vi "Create.vi"(8 "ErrorArray":errorcluster[](array[cluster]), 10 "name or relative path":string="PARTF\\PARTF.ini") -> (0 "ErrorArray":errorcluster[](array[cluster]), 3 "Ref out":refnum<class "Config.lvclass">)   [LabVIEW 2014, in "Config_class.lvlib" / "Config.lvclass"]
uses:
  Config.lvclass
  <vilib>/Utility/sysdir.llb/System Directory Type.ctl
  Typedefs/RootDir.ctl
  Typedefs/Logging.ctl
  Typedefs/eLogLvl.ctl
  Config.lvclass/Config.ctl
  Accessors/Write ConfigFilePath.vi
  Accessors/Write Logging.vi
  Accessors/Write Root Directory.vi
  <vilib>/Utility/config.llb/NI_LVConfig.lvlib
  <userlib>/NIST/NISTErrorLib/NISTErrorLib.lvlib
panel:
  out "before substring":string
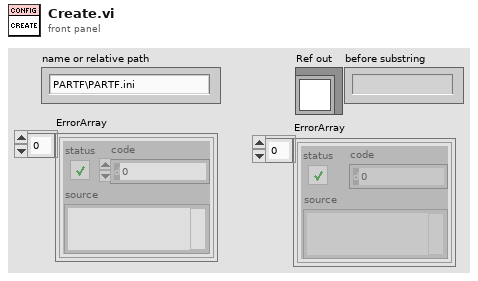
[diagram p1: front panel]
types:
  T1 = typedef "System Directory Type.ctl" = i32
  T2 = typedef "Config_class.lvlib/Config.lvclass/eLogLvl.ctl" = enum16{"Normal", "Verbose", "None"}
  T3 = typedef "Config_class.lvlib/Config.lvclass/Logging.ctl" = cluster{"eLogLvl":T2, "Log File Path":path, "btnLogFile":bool}
  T4 = typedef "Config_class.lvlib/Config.lvclass/RootDir.ctl" = cluster{"pathRootDir":path, "btnOutPath":bool, "OutDir":string, "btnOpenOutputDir":bool, "ScriptDir":string, "btnOpenScriptDir":bool, "TestDir":string, "btnOpenTestDir":bool}
  T5 = cluster{"pathRootDir":path, "OutDir":string, "ScriptDir":string, "TestDir":string}
  T6 = typedef "NI_LVConfig.lvlib/Config Data RefNum.ctl" = refnum<k1>
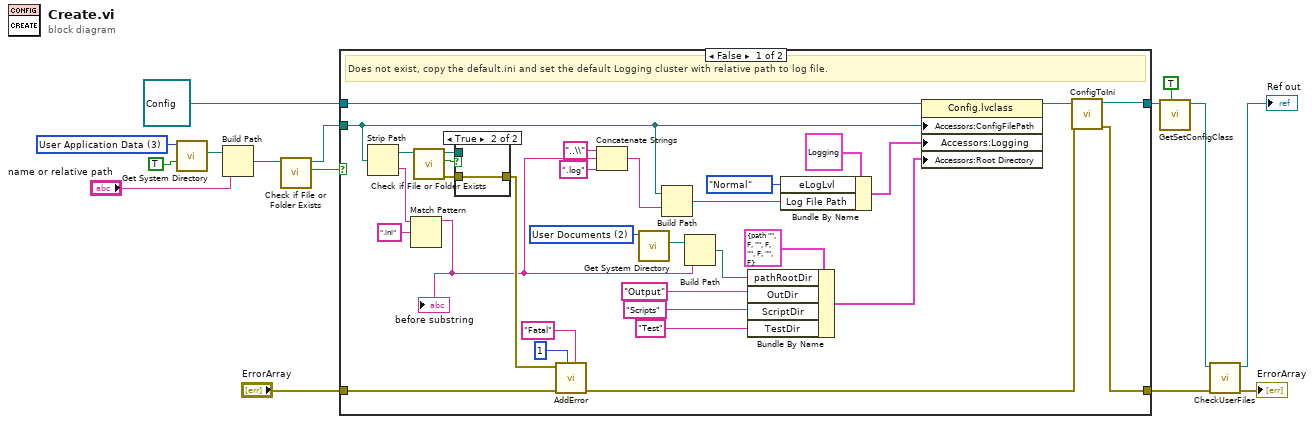
[diagram p0: block diagram]
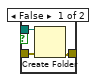
[diagram p2: hidden frame]
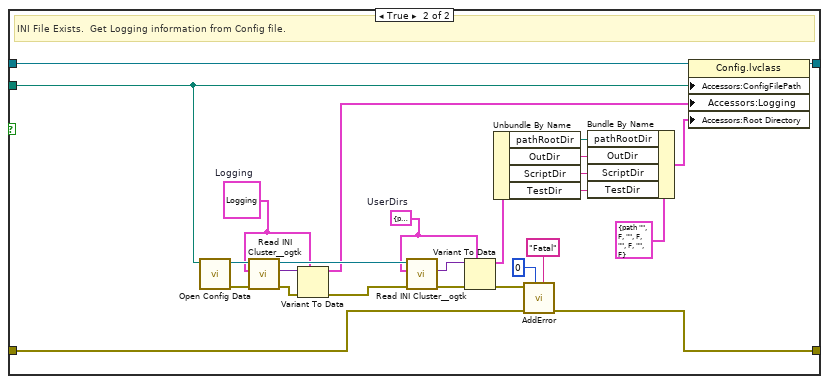
[diagram p3: hidden frame]
diagram:
  w15 = T1 3 items=["User Home"=0, "User Desktop"=1, "User Documents"=2, "User Application Data"=3, "User Preferences"=4, "User Temporary"=5, "Public Documents"=6, "Public Application Data"=7, "Public Preferences"=8, "Public Cache"=13, "System Core Libraries"=9, "System Installed Libraries"=10, "Application Files"=11, "Boot Volume Root"=12] ("system directory type")
  n1 = call <vilib>:"Get System Directory.vi"("create directory if not found? (F)"=TRUE, "system directory type"=w15) -> ("system directory"=w7:path)  [unwired: 9 in]
  n2 = Build Path(base path=w7, name or relative path="name or relative path") -> (appended path=w11:path)
  n3 = call <vilib>:"Check if File or Folder Exists.vi"("path"=w11) -> ("file or folder exists?"=w12:bool, "dup path"=w8:path)  [unwired: 8 in, 1 out]
  n4 = case shown="False" w12 {
    tunnel: w8 -> [w22 w67]
    tunnel: refnum<class "Config.lvclass"> refnum ("Framework.lvlib:Config.lvclass") -> [w47 w77]
    tunnel: [w33 w68] -> w2
    tunnel: "ErrorArray" -> [w31 w64]
    tunnel: [w34 w63] -> w1
    frame False {
      w46 = T1 2 items=["User Home"=0, "User Desktop"=1, "User Documents"=2, "User Application Data"=3, "User Preferences"=4, "User Temporary"=5, "Public Documents"=6, "Public Application Data"=7, "Public Preferences"=8, "Public Cache"=13, "System Core Libraries"=9, "System Installed Libraries"=10, "Application Files"=11, "Boot Volume Root"=12] ("system directory type")
      # "Does not exist, copy the default.ini and set the default Logging cluster with relative path to log file."
      n5 = Strip Path(path=w22) -> (stripped path=w26:path, name=w21:string)
      n6 = Match Pattern(string=w21, regular expression=".ini") -> (before substring=w16:string)  [unwired: 1 in, 3 out]
      "before substring" <- w16
      n7 = call <vilib>:"Check if File or Folder Exists.vi"("path"=w26) -> ("error out"=w23:errorcluster, "file or folder exists?"=w25:bool, "dup path"=w24:path)  [unwired: 8 in]
      n8 = case shown="True" w25 {
        tunnel: [w50 w51] -> w29
        tunnel: w24 -> [w49 _]
        tunnel: w23 -> [w48 w51]
        frame False {
          n9 = Create Folder(path (use dialog)=w49, error in=w48) -> (error out=w50:errorcluster)  [unwired: 1 in, 2 out]
        }
        frame True {
        }
      }
      n10 = call <userlib>:"AddError.vi"("Severity"="Fatal", "Priority"=u8 1, "ErrorArray"=w31, "error in (no error)"=w29) -> ("ErrorArray"=w30:errorcluster[])  [unwired: 6 in, 1 out]
      n11 = Concatenate Strings("..\\" ("string"), w16, ".log" ("string")) -> (w18:string)
      n12 = call <vilib>:"Get System Directory.vi"("system directory type"=w46) -> ("system directory"=w45:path)  [unwired: 10 in]
      n13 = Build Path(base path=w22, name or relative path=w18) -> (appended path=w38:path)
      n14 = Build Path(base path=w45, name or relative path=w16) -> (appended path=w43:path)
      n15 = Bundle By Name(cluster=T4 {"pathRootDir"=path "", "btnOutPath"=FALSE, "OutDir"="", "btnOpenOutputDir"=FALSE, "ScriptDir"="", "btnOpenScriptDir"=FALSE, "TestDir"="", "btnOpenTestDir"=FALSE} ("PARTF Root Directory"), "pathRootDir"=w43, "OutDir"="Output", "ScriptDir"="Scripts", "TestDir"="Test" ("ScriptDir")) -> (w40:T4)
      n16 = Bundle By Name(cluster=T3 {"eLogLvl"=enum."Normal", "Log File Path"=path "C:/Users/gra1/AppData/Local/Framework/Framework.log", "btnLogFile"=FALSE} ("Logging"), "eLogLvl"=eLogLvl."Normal", "Log File Path"=w38) -> (w36:T3)
      n17 = property class="Config.lvclass"(reference=w47, "Accessors:ConfigFilePath"=w22, "Accessors:Logging"=w36, "Accessors:Root Directory"=w40) -> (reference out=w35:refnum<class "Config.lvclass">)  [unwired: 1 in, 1 out]
      n18 = call "ConfigToIni.vi"("Error In"=w30, "ConfigRef"=w35) -> ("Error Out"=w34:errorcluster[], "ConfigRef"=w33:refnum<class "Config.lvclass">)  [unwired: 8 in]
    }
    frame True {
      w60 = T3 {"eLogLvl"=enum."Normal", "Log File Path"=path "C:/Users/gra1/AppData/Local/Framework/Framework.log", "btnLogFile"=FALSE}  # Logging
      w61 = T5 {"pathRootDir"=path "", "OutDir"="", "ScriptDir"="", "TestDir"=""}  # UserDirs
      # "INI File Exists.  Get Logging information from Config file."
      n19 = call <vilib>:"Open Config Data.vi"("configuration file path"=w67) -> ("error out"=w76:errorcluster, "refnum"=w75:T6)  [unwired: 8 in, 1 out]
      n20 = call <userlib>:"Read INI Cluster__ogtk.vi"("error in (no error)"=w76, "INI Fomatted Cluster Type"=w60, "refnum"=w75) -> ("error out"=w74:errorcluster, "INI Fomatted Cluster"=w73:variant, "dup refnum"=w72:T6)  [unwired: 4 in, 2 out]
      n21 = Variant To Data(error in=w74, type=w60, Variant=w73) -> (data=w59:T3, error out=w71:errorcluster)
      n22 = call <userlib>:"Read INI Cluster__ogtk.vi"("error in (no error)"=w71, "INI Fomatted Cluster Type"=w61, "refnum"=w72) -> ("error out"=w70:errorcluster, "INI Fomatted Cluster"=w69:variant)  [unwired: 4 in, 3 out]
      n23 = Variant To Data(error in=w70, type=w61, Variant=w69) -> (data=w58:T5, error out=w62:errorcluster)
      n24 = Unbundle By Name(w58) -> ("pathRootDir"=w56:path, "OutDir"=w55:string, "ScriptDir"=w54:string, "TestDir"=w53:string)
      n25 = call <userlib>:"AddError.vi"("Severity"="Fatal", "Priority"=u8 0, "ErrorArray"=w64, "error in (no error)"=w62) -> ("ErrorArray"=w63:errorcluster[])  [unwired: 6 in, 1 out]
      n26 = Bundle By Name(cluster=T4 {"pathRootDir"=path "", "btnOutPath"=FALSE, "OutDir"="", "btnOpenOutputDir"=FALSE, "ScriptDir"="", "btnOpenScriptDir"=FALSE, "TestDir"="", "btnOpenTestDir"=FALSE} ("PARTF Root Directory"), "pathRootDir"=w56, "OutDir"=w55, "ScriptDir"=w54, "TestDir"=w53) -> (w52:T4)
      n27 = property class="Config.lvclass"(reference=w77, "Accessors:ConfigFilePath"=w67, "Accessors:Logging"=w59, "Accessors:Root Directory"=w52) -> (reference out=w68:refnum<class "Config.lvclass">)  [unwired: 1 in, 1 out]
    }
  }
  n28 = call "GetSetConfigClass.vi"("Set (f)"=TRUE, "Ref in"=w2) -> ("Ref out"=w5:refnum<class "Config.lvclass">)  [unwired: 9 in]
  n29 = call "CheckUserFiles.vi"("ErrorArray"=w1, "Config in"=w5) -> ("ErrorArray"=→"ErrorArray":errorcluster[], "Config out"=→"Ref out":refnum<class "Config.lvclass">)  [unwired: 8 in]
